vi "Watch_Directory_Snap.vi"() -> ()   [LabVIEW 2015]
uses:
  <userlib>/caLab/Private/Get_PV-1D.vi
panel:
  out "concatenated string 2":string
  in  "string 2":string="P:\\bl13-0\\bl13-2\\dt_SES100\\"
  in  "OK Button":bool
  in  "ELOG":string
  out "path":path
  out "file path 2":path=path "S:/"
  in  "Ring":u16(ring) items=["SES-100", "R3000"]
  out "spreadsheet string":string
  out "PV Names (dup)":string[](array[string])
  out "PV2ELOG":string
  out "concatenated string":string
  out "standard error":string
  out "standard output":string
  out "x = y?":bool
  out "File Name 1":string
  in  "Filter":string
  in  "stop":bool
  out "File Name 0":string
  in  "Path":path=path "D:/Documents and Settings/Customer Education/My Documents"
  # "Set a folder to watch using the\nPath control. You can also\nset a filter for a certain type\nof file to watch for (such as\n*.bmp). Then run the\nexample. Whenever you create\na new file in that directory that\nmatches the filter, New File Name\nwill update to let you know the\nnew file name."
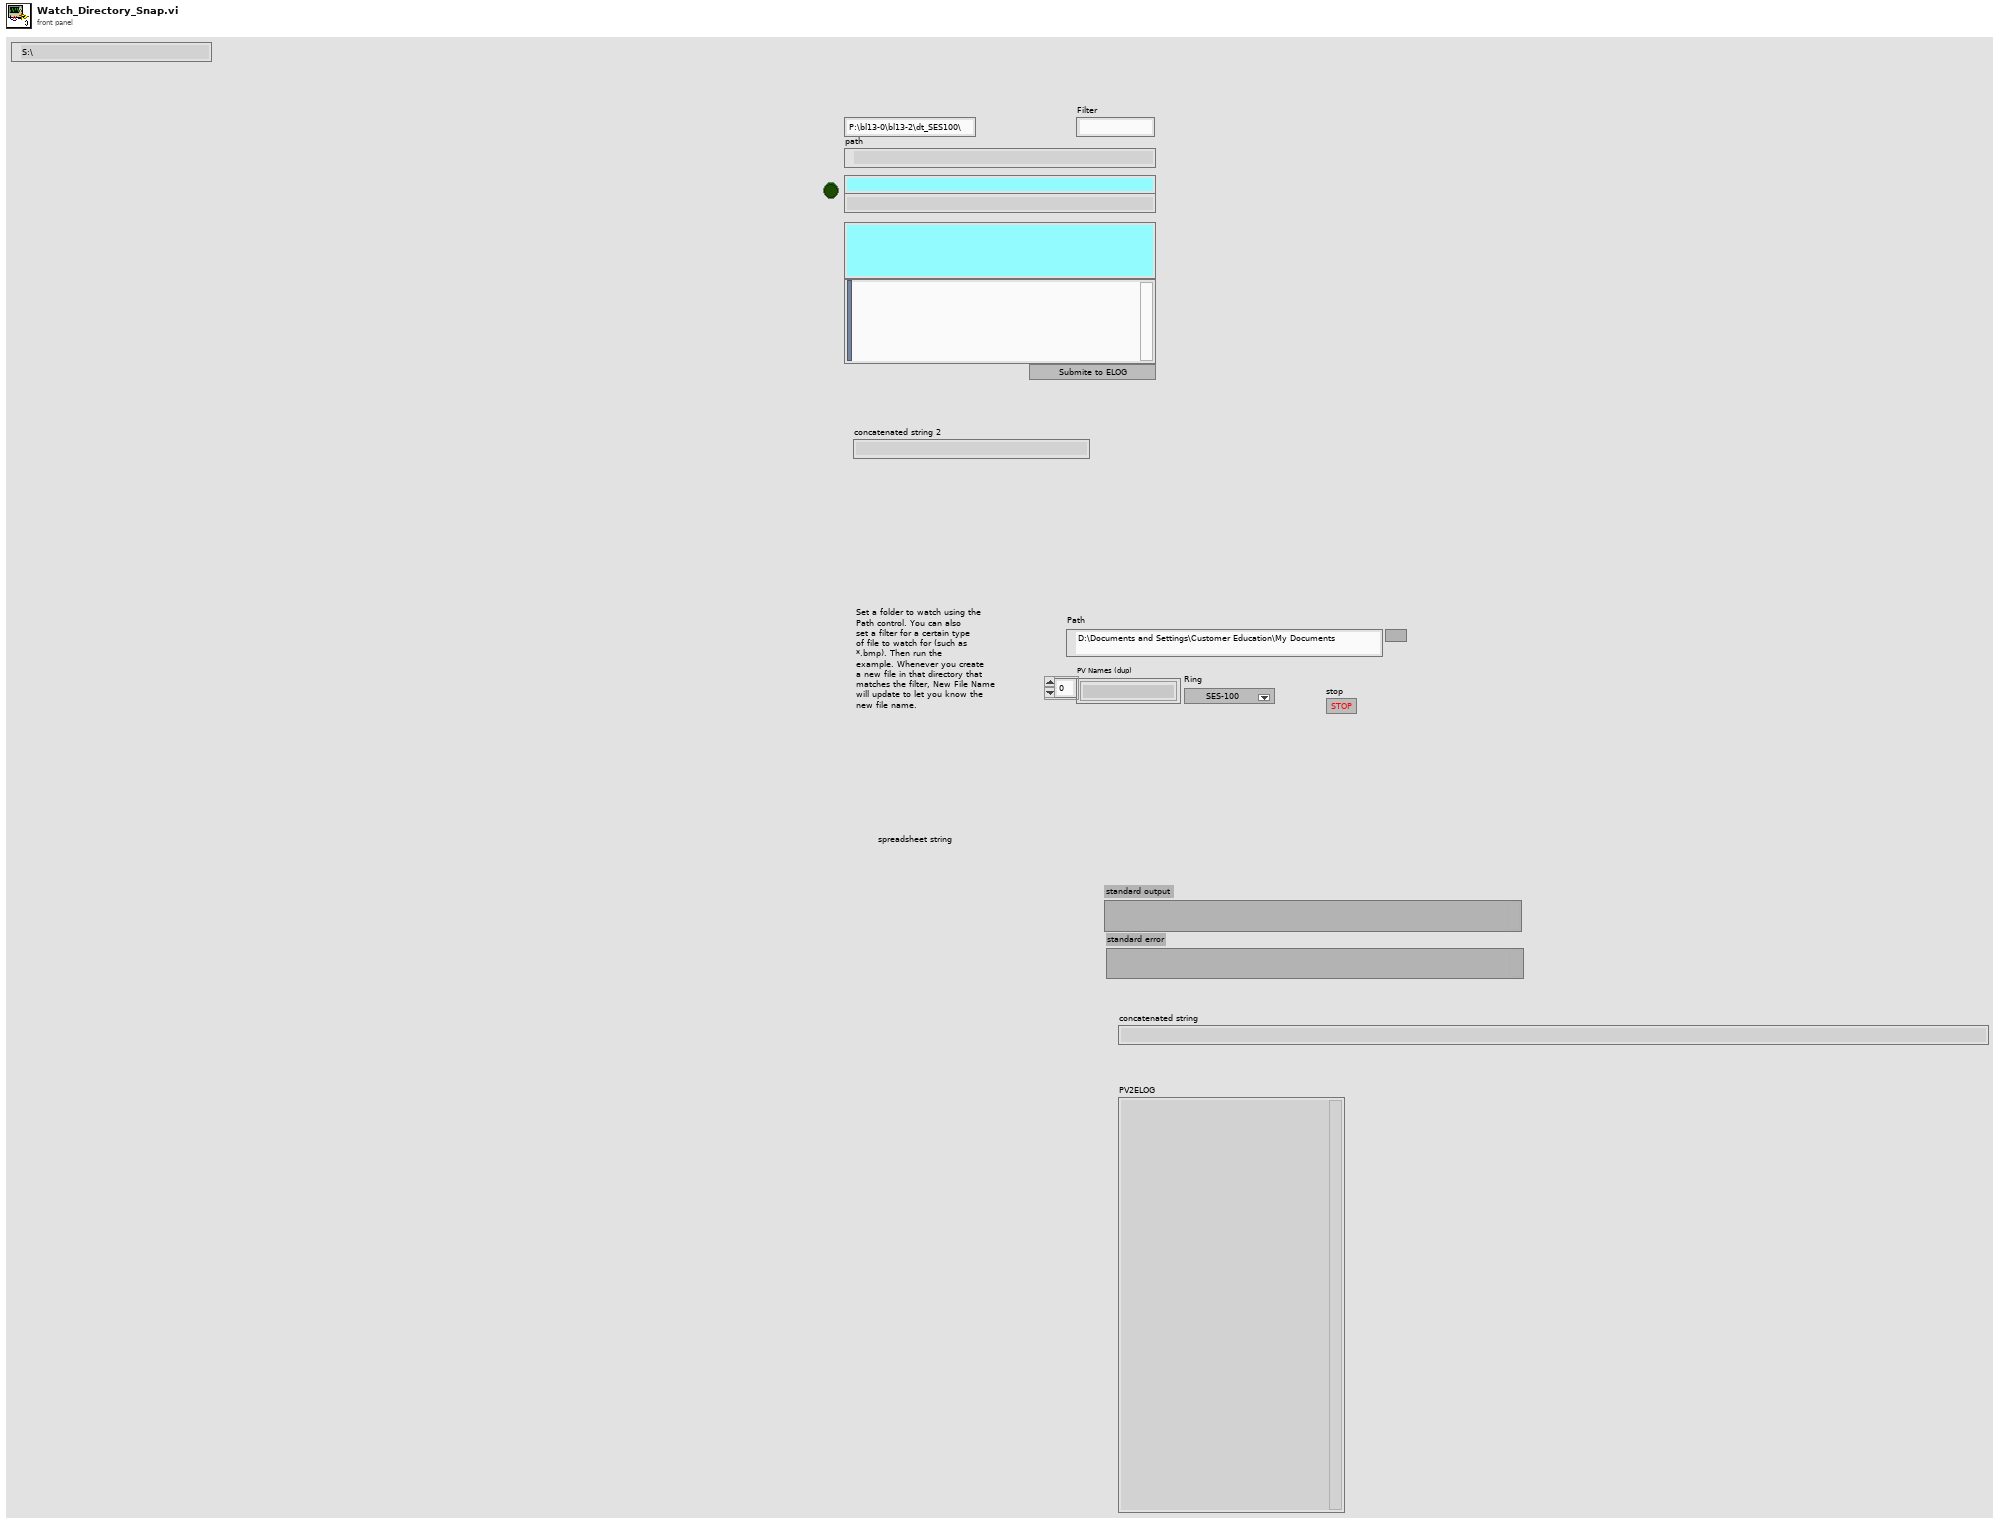
[diagram p1: front panel]
types:
  T1 = enum16{"open", "replace", "create", "open or create", "replace or create", "replace or create with confirmation"}
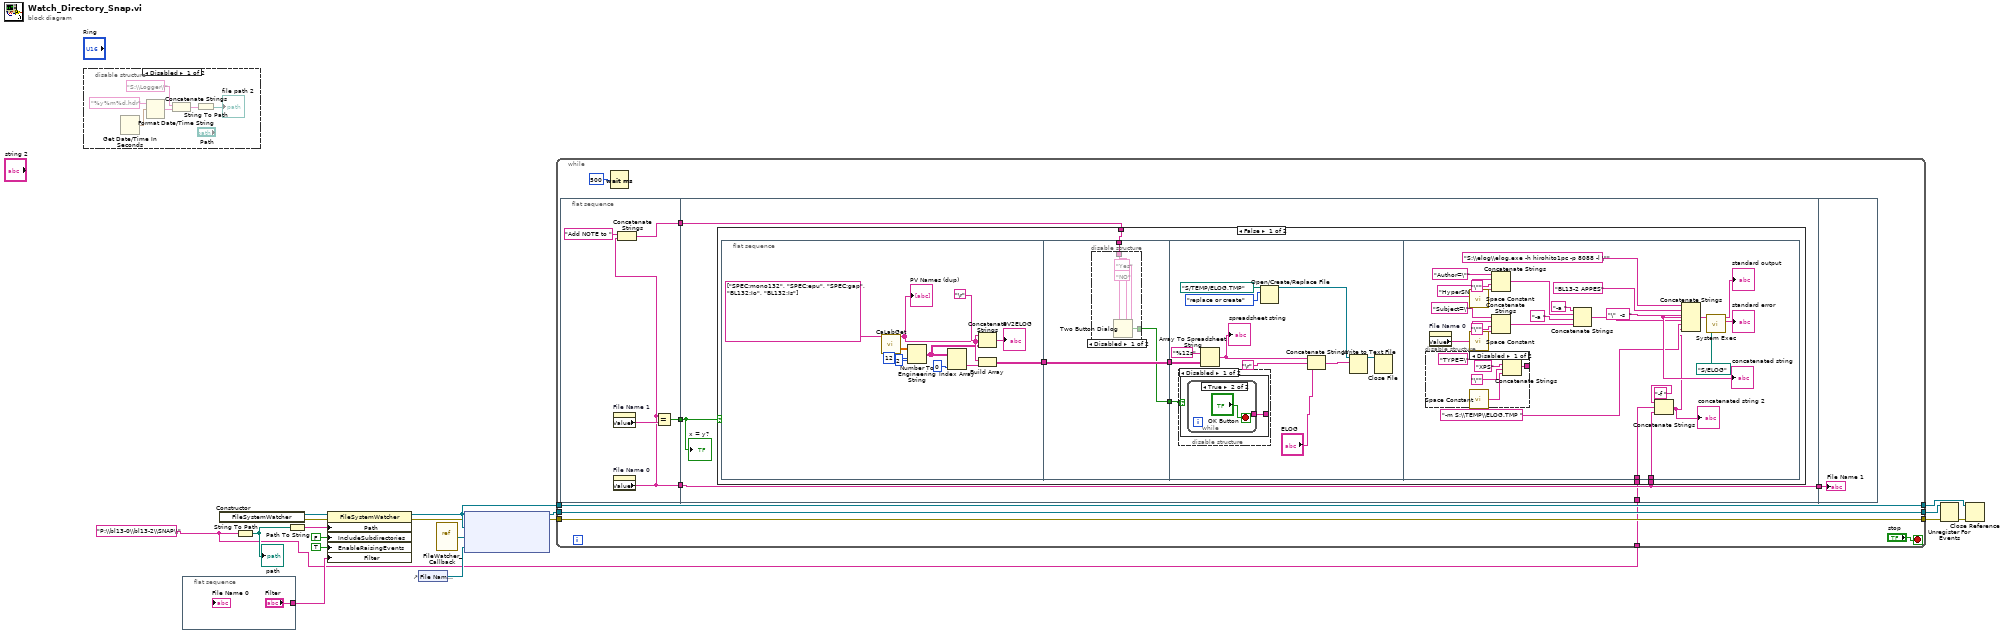
[diagram p0: block diagram]
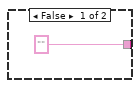
[diagram p4: hidden frame]
diagram:
  w2 = "P:\\bl13-0\\bl13-2\\SNAP\\" ("string")
  n1 = disable-structure shown="Disabled" {
    frame Disabled {
      n2 = Get Date/Time In Seconds() -> (seconds since 1Jan1904=w24:timestamp)
      n3 = Format Date/Time String(time format string (%c)="%y%m%d.hdr", seconds (now)=w24) -> (date/time string=w21:string)  [unwired: 1 in]
      n4 = Concatenate Strings("S:\\Logger\\", w21) -> (w20:string)
      n5 = String To Path(string=w20) -> (path=→"file path 2":path)
    }
    frame Enabled {
    }
  }
  n6 = flat-sequence {
    tunnel: ["Filter"] -> w5
    frame #0 {
    }
  }
  n7 = constructor class="FileSystemWatcher"() -> (reference out=w18:refnum<k24>, error out=w10:errorcluster)  [unwired: 3 in, 1 out]
  n8 = String To Path(string=w2) -> (path=w3:path)
  "path" <- w3
  n9 = Path To String(path=w3) -> (string=w1:string)
  n10 = property class="FileSystemWatcher"(reference=w18, error in=w10, "Path"=w1, "IncludeSubdirectories"=FALSE, "EnableRaisingEvents"=TRUE, "Filter"=w5) -> (reference out=w13:refnum<k24>, error out=w9:errorcluster)
  n11 = control-ref of="File Name 0"() -> (w4:refnum<vi>)
  n12 = vi-ref "FileWatcher_Callback.vi"() -> ("vi reference"=w16:refnum<vi>)
  n13 = node(w9, w13, w16, w4) -> (w14:refnum<k27>, w7:errorcluster)  [unwired: 1 in]
  n14 = while {
    tunnel: [w34] -> w15
    tunnel: w14 -> [w34]
    tunnel: [w33] -> w11
    tunnel: w13 -> [w33]
    tunnel: [w32] -> w8
    tunnel: w7 -> [w32]
    tunnel: w2 -> [w26]
    stop <- "stop" stop-if-true
    n15 = flat-sequence {
      tunnel: [w37] -> w30
      tunnel: [w39] -> w28
      tunnel: [w36] -> w27
      tunnel: w30 -> [w42]
      tunnel: [w42] -> w29
      tunnel: w28 -> [w44]
      tunnel: w27 -> [w43]
      tunnel: w26 -> [w41]
      tunnel: w29 -> [w115]
      frame #0 {
        n16 = property on="File Name 1" class="Str"() -> ("Value"=w40:string)  [unwired: 2 in, 2 out]
        n17 = property on="File Name 0" class="Str"() -> ("Value"=w37:string)  [unwired: 2 in, 2 out]
        n18 = Concatenate Strings("Add NOTE to " ("string"), w37) -> (w36:string)
        n19 = Equal?(x=w37, y=w40) -> (x = y?=w39:bool)
      }
      frame #1 {
        n20 = case shown="False" w44 {
          tunnel: w43 -> [w48 _]
          tunnel: w42 -> [w46 _]
          tunnel: w41 -> [w45 _]
          frame False {
            n21 = flat-sequence {
              tunnel: [w53] -> w49
              tunnel: [w64] -> w50
              tunnel: w49 -> [w64]
              tunnel: w48 -> [w63]
              tunnel: [w62] -> w47
              tunnel: w50 -> [w74]
              tunnel: w47 -> [w70]
              tunnel: w46 -> [w90]
              tunnel: w45 -> [w89]
              frame #0 {
                n22 = call-poly <userlib>:"CaLabGet.vi"("PV Names"=string[] ["SPEC:mono132", "SPEC:epu", "SPEC:gap", "BL132:Io", "BL132:Is"]) -> ("PV Names (dup)"=w57:string[], "Value Array (number)"=w59:dbl[][])  [unwired: 8 in, 5 out]
                "PV Names (dup)" <- w57
                n23 = Number To Engineering String(2:i16 2 ("precision (6)"), 3:i16 12 ("width (-)"), 4:w59) -> (0:w55:string[][])  [unwired: 1 in]
                n24 = Index Array(array=w55, index (col)=0) -> (element=w54:string[])  [unwired: 1 in]
                n25 = Concatenate Strings(w57, "\r", w55) -> (→"PV2ELOG":string)
                n26 = Build Array(w57, w54) -> (w53:string[][])
              }
              frame #1 {
                n27 = disable-structure shown="Disabled" {
                  disable-tunnel: w63 -> [w68 _]
                  disable-tunnel: [w65 _] -> w62
                  frame Disabled {
                    n28 = Two Button Dialog(message=w68, 1:"NO" ("F button name (\"Cancel\")"), 2:"Yes" ("T button name (\"OK\")")) -> (T button?=w65:bool)
                  }
                  frame Enabled {
                  }
                }
              }
              frame #2 {
                n29 = disable-structure shown="Disabled" {
                  disable-tunnel: w70 -> [w80 _]
                  frame Disabled {
                    n30 = case shown="True" w80 {
                      tunnel: ["" ("ELOG") w82] -> _
                      frame False {
                      }
                      frame True {
                        n31 = while {
                          tunnel: w82 -> [w84]
                          stop <- "OK Button" stop-if-true
                        }
                      }
                    }
                  }
                  frame Enabled {
                  }
                }
                n32 = Array To Spreadsheet String(array=w74, 3:"%12s" ("format string")) -> (spreadsheet string=w72:string)  [unwired: 1 in]
                "spreadsheet string" <- w72
                n33 = Open/Create/Replace File(file path (use dialog)=path "S:/TEMP/ELOG.TMP", operation (0:open)=T1."replace or create") -> (refnum out=w79:refnum<file>)  [unwired: 4 in, 2 out]
                n34 = Concatenate Strings(w72, "\r", "ELOG") -> (w71:string)
                n35 = Write to Text File(file (use dialog)=w79, text=w71) -> (refnum out=w78:refnum<file>)  [unwired: 2 in, 2 out]
                n36 = Close File(refnum=w78) -> ()  [unwired: 1 in, 2 out]
              }
              frame #3 {
                n37 = disable-structure shown="Disabled" {
                  disable-tunnel: [w110 _] -> _
                  frame Disabled {
                    n38 = call <vilib>:"Space Constant.vi"() -> ("String"=w111:string)
                    n39 = Concatenate Strings("TYPE=\"" ("string"), "XPS", "\"" ("string"), w111) -> (w110:string)
                  }
                  frame Enabled {
                  }
                }
                n40 = property on="File Name 0" class="Str"() -> ("Value"=w91:string)  [unwired: 2 in, 2 out]
                n41 = call <vilib>:"Space Constant.vi"() -> ("String"=w97:string)
                n42 = call <vilib>:"Space Constant.vi"() -> ("String"=w88:string)
                n43 = Concatenate Strings("Author=\"" ("string"), "HyperSNAP", "\"" ("string"), w97) -> (w95:string)
                n44 = Concatenate Strings("Subject=\"" ("string"), w91, "\"" ("string"), w88) -> (w93:string)
                n45 = Concatenate Strings("-a ", w95, "-a " ("string"), w93) -> (w94:string)
                n46 = Concatenate Strings("-f " ("string"), w89, w90) -> (w85:string)
                "concatenated string 2" <- w85
                n47 = Concatenate Strings("S:\\elog\\elog.exe -h hirohito1pc -p 8088 -l \"" ("command line"), "BL13-2 APPES", "\"  -s  " ("command line"), w94, "-m S:\\TEMP\\ELOG.TMP " ("string"), w85) -> (w105:string)
                "concatenated string" <- w105
                n48 = call <vilib>:"System Exec.vi"("working directory"=path "S:/ELOG", "command line"=w105) -> ("standard error"=→"standard error":string, "standard output"=→"standard output":string)  [unwired: 6 in, 2 out]
              }
            }
          }
          frame True {
          }
        }
        "x = y?" <- w44
      }
      frame #2 {
        "File Name 1" <- w115
      }
    }
    n49 = Wait (ms)(milliseconds to wait=u32 500) -> ()  [unwired: 1 out]
  }
  n50 = Unregister For Events(event registration refnum=w15, error in=w8) -> (error out=w12:errorcluster)
  n51 = Close Reference(reference=w11, error in (no error)=w12) -> ()  [unwired: 1 out]
